vi "Set_Setting_USB7855R.vi"(5 "ChangeonFly":T3, 8 "SettingsCluster":T1={"Sample Rate (us)"=1, "Samples Per Data Point (int, power of 2)"=1000, "DistanceToBulk (um)"=-1.0, "HoldTimeScaler"=1, "SaveData"=TRUE, "DistanceToBulk (um) 2"=-1.0, "DistanceToBulk (um) 3"=-1.0}, 9 "VelScallerCluster":T2, 11 "FPGA VI Reference Out":refnum<k20>) -> (0 "FPGAAccumulatorLength_inpowersof2":i16)   [LabVIEW 2023]
uses:
  TypeDefs/ChangeOnFly.ctl
  TypeDefs/VelScallerCluster.ctl
  TypeDefs/Settings.ctl
  User_Vi/Settings.vi
  <vilib>/Utility/error.llb/Error Cluster From Error Code.vi
  <vilib>/rvi/errors/niLvFpgaAdjustHostInterfaceError.vi
  <vilib>/rvi/interface/nirviReadWriteControl/nirviReadWriteControl.xnode
  NiFpgaLv.dll
  <vilib>/rvi/interface/Simulation/niFpgaSimulationCallBeginRW.vi
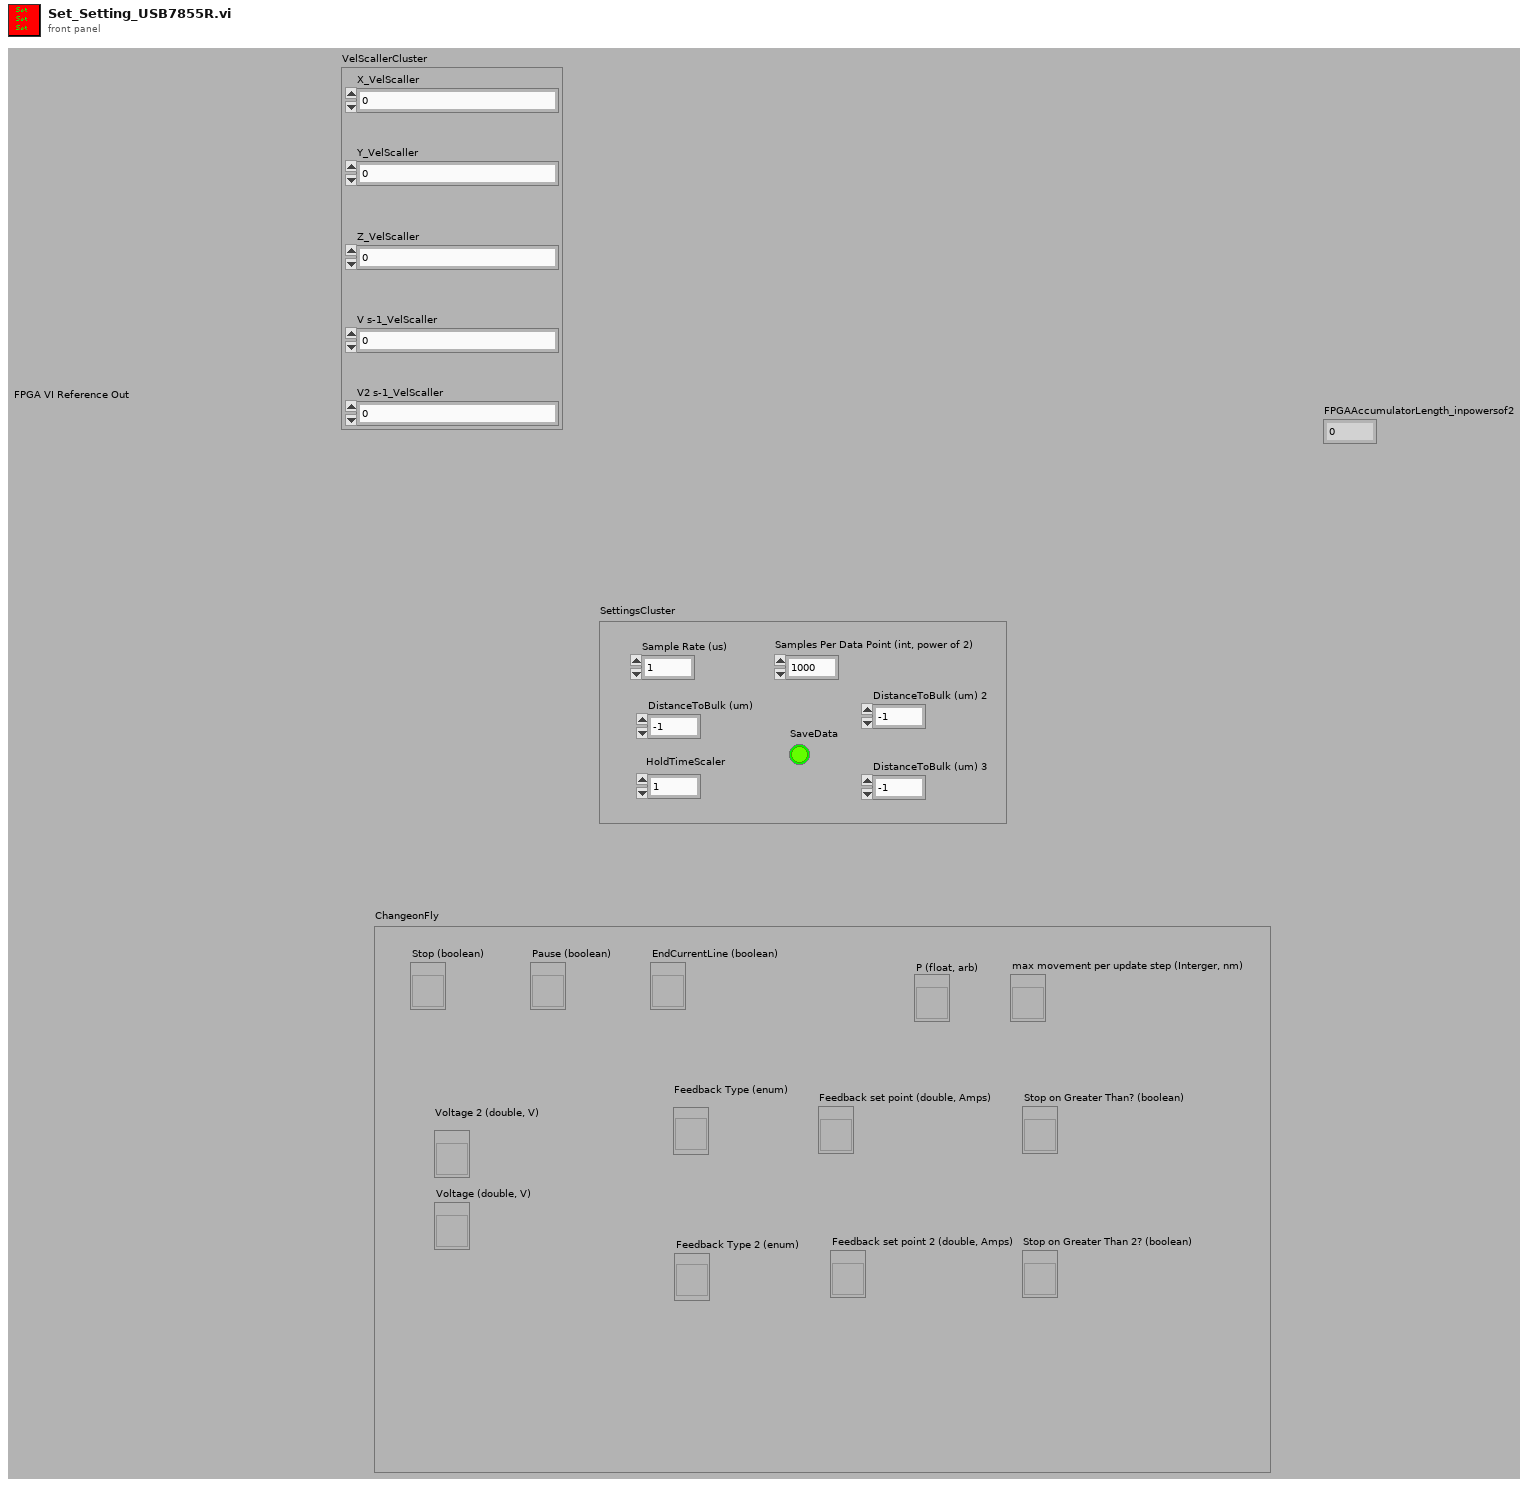
[diagram p1: front panel]
types:
  T1 = typedef "Settings.ctl" = cluster{"Sample Rate (us)":u32, "Samples Per Data Point (int, power of 2)":i16, "DistanceToBulk (um)":dbl, "HoldTimeScaler":u64, "SaveData":bool, "DistanceToBulk (um) 2":dbl, "DistanceToBulk (um) 3":dbl}
  T2 = typedef "VelScallerCluster.ctl" = cluster{"X_VelScaller":i32, "Y_VelScaller":i32, "Z_VelScaller":i32, "V s-1_VelScaller":i32, "V2 s-1_VelScaller":i32}
  T3 = typedef "ChangeOnFly.ctl" = cluster{"Stop (boolean)":refnum<vi>, "Pause (boolean)":refnum<vi>, "EndCurrentLine (boolean)":refnum<vi>, "max movement per update step (Interger, nm)":refnum<vi>, "P (float, arb)":refnum<vi>, "Feedback set point (double, Amps)":refnum<vi>, "Voltage (double, V)":refnum<vi>, "Feedback set point 2 (double, Amps)":refnum<vi>, "Stop on Greater Than 2? (boolean)":refnum<vi>, "Stop on Greater Than? (boolean)":refnum<vi>, "Voltage 2 (double, V)":refnum<vi>, "Feedback Type (enum)":refnum<vi>, "Feedback Type 2 (enum)":refnum<vi>}
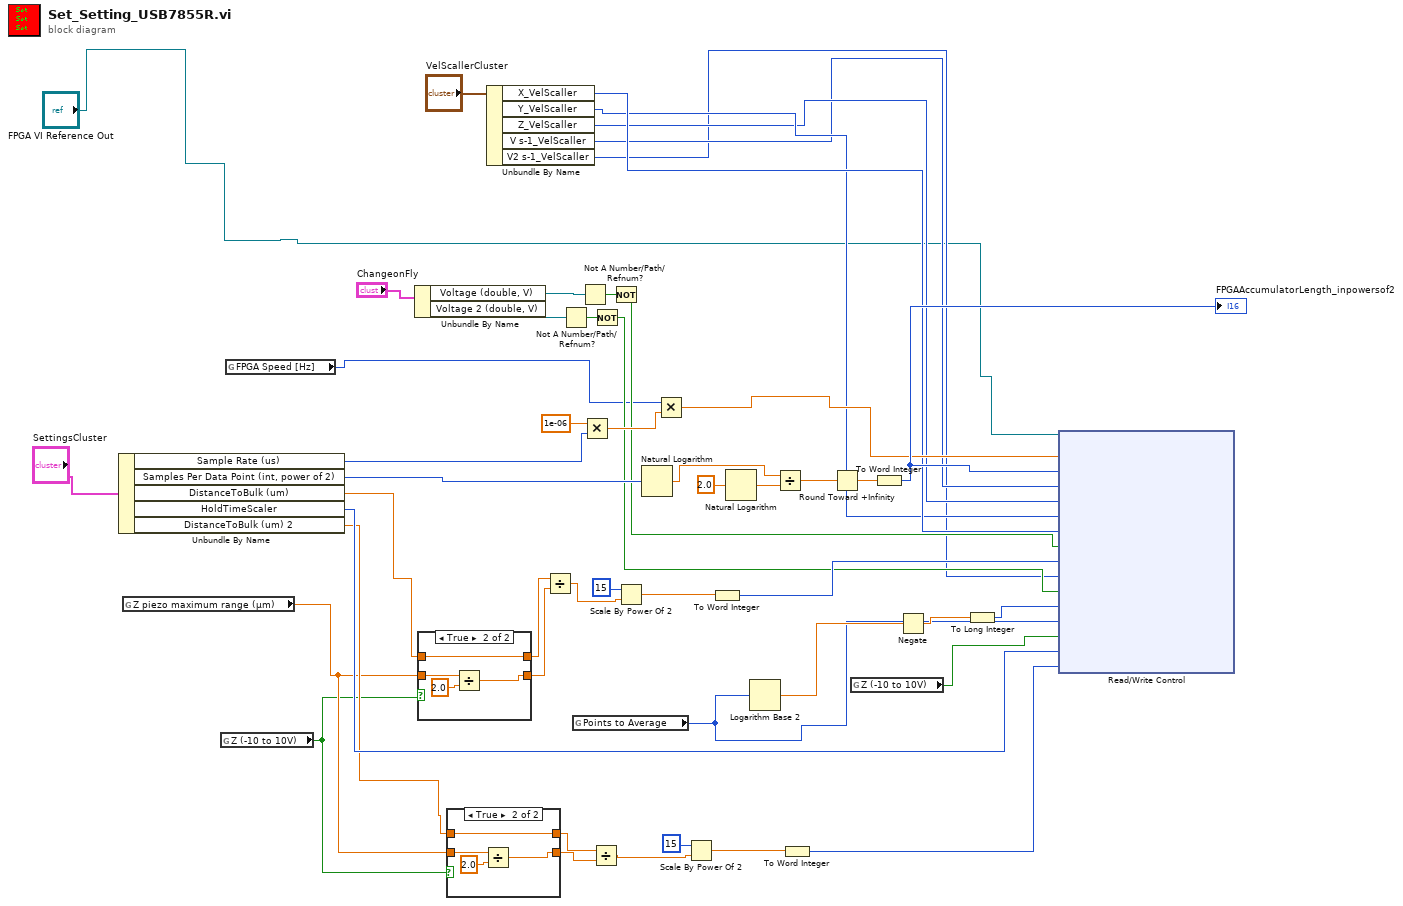
[diagram p0: block diagram]
diagram:
  n1 = Unbundle By Name("SettingsCluster") -> ("Sample Rate (us)"=w39:u32, "Samples Per Data Point (int, power of 2)"=w48:i16, "DistanceToBulk (um)"=w25:dbl, "HoldTimeScaler"=w14:u64, "DistanceToBulk (um) 2"=w8:dbl)
  n2 = global read "Settings.vi" "Z piezo maximum range (µm)"() -> (w7:dbl)
  n3 = global read "Settings.vi" "Z (-10 to 10V)"() -> (w6:bool)
  n4 = global read "Settings.vi" "FPGA Speed [Hz]"() -> (w13:i64)
  n5 = Unbundle By Name("ChangeonFly") -> ("Voltage (double, V)"=w33:refnum<vi>, "Voltage 2 (double, V)"=w29:refnum<vi>)
  n6 = case shown="True" w6 {
    tunnel: w25 -> [w51 w52]
    tunnel: [w51 w52] -> w24
    tunnel: [w50 w53] -> w23
    tunnel: w7 -> [w50 w54]
    frame False {
    }
    frame True {
      n7 = Divide(x=w54, y=2.0) -> (x/y=w53:dbl)
    }
  }
  n8 = case shown="True" w6 {
    tunnel: w8 -> [w57 w58]
    tunnel: [w57 w58] -> w10
    tunnel: [w56 w59] -> w9
    tunnel: w7 -> [w56 w60]
    frame False {
    }
    frame True {
      n9 = Divide(x=w60, y=2.0) -> (x/y=w59:dbl)
    }
  }
  n10 = Unbundle By Name("VelScallerCluster") -> ("X_VelScaller"=w20:i32, "Y_VelScaller"=w19:i32, "Z_VelScaller"=w18:i32, "V s-1_VelScaller"=w17:i32, "V2 s-1_VelScaller"=w16:i32)
  n11 = Divide(x=w24, y=w23) -> (x/y=w40:dbl)
  n12 = Not A Number/Path/Refnum?(number/path/refnum=w29) -> (NaN/Path/Refnum?=w30:bool)
  n13 = global read "Settings.vi" "Points to Average"() -> (w12:u16)
  n14 = Not A Number/Path/Refnum?(number/path/refnum=w33) -> (NaN/Path/Refnum?=w34:bool)
  n15 = Multiply(x=1e-06, y=w39) -> (x*y=w38:dbl)
  n16 = Divide(x=w10, y=w9) -> (x/y=w3:dbl)
  n17 = Not(x=w30) -> (.not. x?=w28:bool)
  n18 = Not(x=w34) -> (.not. x?=w32:bool)
  n19 = Scale By Power Of 2(n=15, x=w40) -> (x*2^n=w42:dbl)
  n20 = Natural Logarithm(1:w48) -> (0:w43:dbl)
  n21 = Multiply(x=w13, y=w38) -> (x*y=w36:dbl)
  n22 = Scale By Power Of 2(n=15, x=w3) -> (x*2^n=w5:dbl)
  n23 = To Word Integer(number=w42) -> (16bit integer=w31:i16)
  n24 = Natural Logarithm(1:2.0 ("x")) -> (0:w44:dbl)
  n25 = Logarithm Base 2(1:w12) -> (0:w27:dbl)
  n26 = Divide(x=w43, y=w44) -> (x/y=w46:dbl)
  n27 = To Word Integer(number=w5) -> (16bit integer=w2:i16)
  n28 = Round Toward +Infinity(x=w46) -> (ceil(x): smallest int >= x=w47:dbl)
  n29 = global read "Settings.vi" "Z (-10 to 10V)"() -> (w11:bool)
  n30 = To Word Integer(number=w47) -> (16bit integer=w49:i16)
  "FPGAAccumulatorLength_inpowersof2" <- w49
  n31 = Negate(x=w27) -> (-x=w22:dbl)
  n32 = To Long Integer(number=w22) -> (32bit integer=w26:i32)
  n33 = xnode ("Read/Write Control")("FPGA VI Reference In"="FPGA VI Reference Out", "Buffer Loop Wait Time (tICKS)"=w36, "2^(-n)"=w49, "ExpandVelScaller V"=w17, "ExpandVelScaller Z"=w18, "ExpandVelScaller Y"=w19, "ExpandVelScaller X"=w20, "Change V on Fly"=w32, "DistanceToBulk"=w31, "ExpandVelScaller V2"=w16, "Change V on Fly 2"=w28, "P2AvgMinus"=w26, "P2AvgWhole"=w12, "Z_axis_-10Vto10V"=w11, "HoldTimerScale"=w14, "DistanceToBulk 2"=w2) -> ()  [unwired: 1 in, 2 out]
